vi "setDelayExposureTime.vi"(8 "error in (no error)":errorcluster, 9 "delay_time_s":dbl, 10 "exposure_time_s":dbl, 11 "Camera in":refnum<class "Camera.lvclass">) -> (0 "error out":errorcluster, 3 "Camera out":refnum<class "Camera.lvclass">)   [LabVIEW 2019, in "Camera.lvclass"]
doc: "Sets the delay and exposure time of the camera, in seconds. The values for the underlying pco.sdk function\nPCO_SetDelayExposureTime.vi will be calculated automatically."
uses:
  Camera.lvclass
  Camera.lvclass/Camera.ctl
  pco.sdk/TimingControl/TimingControl.lvlib
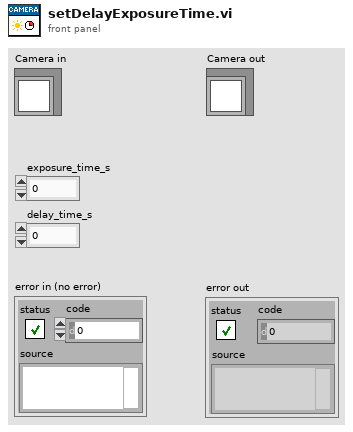
[diagram p1: front panel]
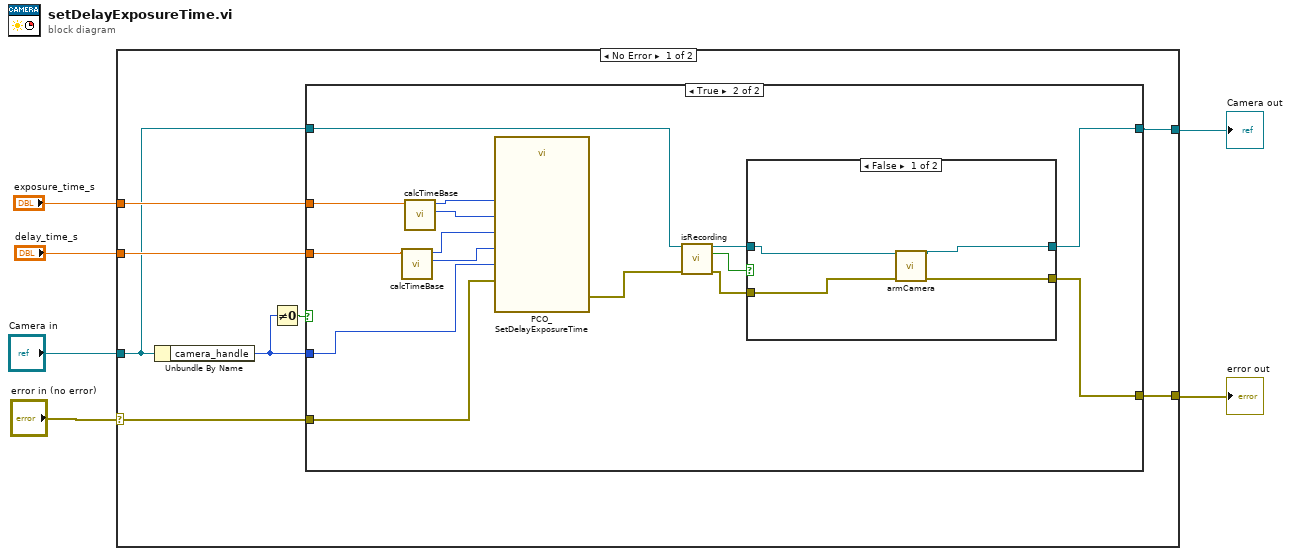
[diagram p0: block diagram]
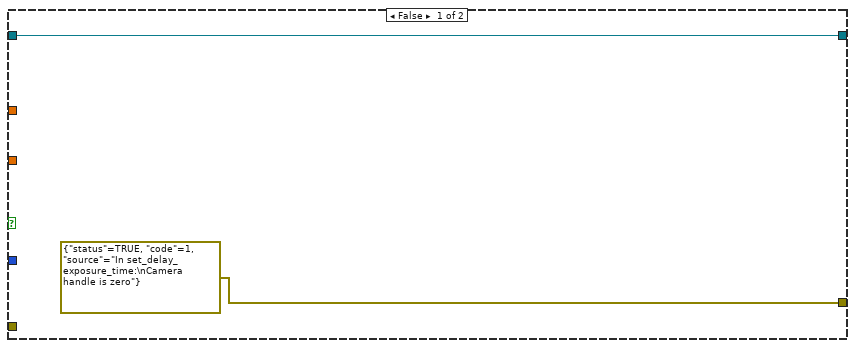
[diagram p2: hidden frame]
diagram:
  n1 = case shown="No Error" "error in (no error)" {
    selector: "error in (no error)" -> [w11 w39]
    tunnel: [w9 w39] -> w5
    tunnel: [w7 w38] -> w3
    tunnel: "Camera in" -> [w8 w38]
    tunnel: "exposure_time_s" -> [w12 _]
    tunnel: "delay_time_s" -> [w10 _]
    frame No Error {
      n2 = Unbundle By Name(w8) -> ("camera_handle"=w13:u64)
      n3 = Not Equal To 0?(x=w13) -> (x != 0?=w14:bool)
      n4 = case shown="True" w14 {
        tunnel: [errorcluster {"status"=TRUE, "code"=1, "source"="In set_delay_exposure_time:\nCamera handle is zero"} ("error constant") w21] -> w9
        tunnel: w13 -> [_ w30]
        tunnel: w11 -> [_ w31]
        tunnel: w12 -> [_ w29]
        tunnel: w10 -> [_ w19]
        tunnel: w8 -> [w15 w26]
        tunnel: [w15 w20] -> w7
        frame False {
        }
        frame True {
          n5 = call "calcTimeBase.vi"("time"=w19) -> ("base_calculated"=w17:u16, "time_calculated"=w18:u32)  [unwired: 9 in]
          n6 = call "calcTimeBase.vi"("time"=w29) -> ("base_calculated"=w27:u16, "time_calculated"=w28:u32)  [unwired: 9 in]
          n7 = call "PCO_SetDelayExposureTime.vi"("wTimeBaseExposure"=w27, "wTimeBaseDelay"=w17, "error in (no error)"=w31, "dwExposure"=w28, "dwDelay"=w18, "ph"=w30) -> ("error out"=w25:errorcluster)  [unwired: 3 in, 2 out]
          n8 = call-dynamic "isRecording.vi"("Camera in"=w26, "error in (no error)"=w25) -> ("Camera out"=w23:refnum<class "Camera.lvclass">, "recording"=w24:bool, "error out"=w22:errorcluster)  [unwired: 11 in]
          n9 = case shown="False" w24 {
            tunnel: w23 -> [w33 w37]
            tunnel: [w32 w37] -> w20
            tunnel: w22 -> [w35 w36]
            tunnel: [w34 w36] -> w21
            frame False {
              n10 = call-dynamic "armCamera.vi"("Camera in"=w33, "error in (no error)"=w35) -> ("Camera out"=w32:refnum<class "Camera.lvclass">, "error out"=w34:errorcluster)  [unwired: 12 in]
            }
            frame True {
            }
          }
        }
      }
    }
    frame Error {
    }
  }
  "error out" <- w5
  "Camera out" <- w3
